vi "test_Bitfile Reload_Simple Scalar to Speciality IO Data type Change.vi"(8 "error in (no error)":errorcluster, 11 "TestCase in":refnum<class "FPGA Addon Bitfile Reload Unit Tests.lvclass">=refnum) -> (0 "error out":errorcluster, 3 "TestCase out":refnum<class "FPGA Addon Bitfile Reload Unit Tests.lvclass">)   [LabVIEW 2026, in "FPGA Addon Bitfile Reload Unit Tests.lvclass"]
uses:
  FPGA Addon Bitfile Reload Unit Tests.lvclass
  APIs/Scripting API/TypeDefs/Output Scalar Data.ctl
  APIs/Scripting API/Scripting API.lvlib
  FPGA Addon Test Class/FPGA Addon Test Class.lvclass
  Addon/Addon System Explorer/FPGA Addon System Explorer.lvlib
  APIs/Scripting API/Public/Bitfile Resources/Import Bitfile Scalars (Instances)/Import Scalars - all.vi
  Addon/Addon Shared/Types/FPGA Addon Data Type.ctl
  Addon/Addon Shared/FPGA Addon Shared.lvlib
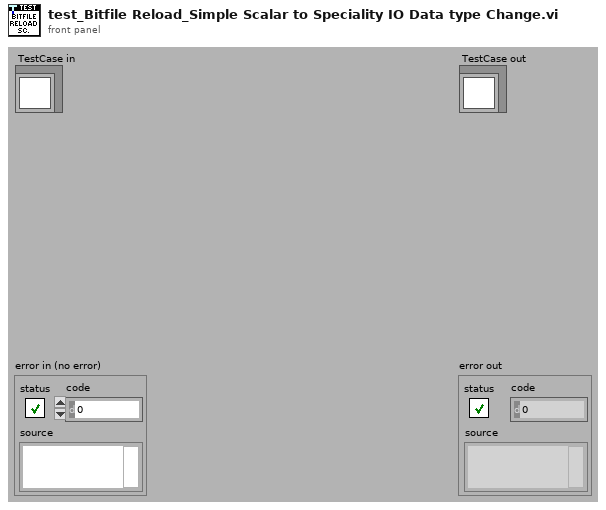
[diagram p1: front panel]
types:
  T1 = typedef "Scripting API.lvlib/Output Scalar Data.ctl" = cluster{"Bitfile Name":string, "SysDef Channel Name":string, "Imported":bool, "Data Type":T2}
  T2 = typedef "FPGA Addon Shared.lvlib/FPGA Addon Data Type.ctl" = enum8{"<Null>", "I8", "I16", "I32", "I64", "U8", "U16", "U32", "U64", "SGL", "Boolean", "Analog PWM In Settings", "Analog PWM In", "Digital PWM In Settings", "Digital PWM In", "Digital PWM Out", "Sine Out", "FXP", "FXP+/-24.5", "FXP+/-16.5", "FXP+/-32.8", "FXP+/-64.32", "FXP+/-16.7", "FXP+/-20.5", "FXP+/-27.5", "FXP+/-32.16", "FXP+16.3", "FXP+18.3", "Digital Static In", "Digital Static Out", "Digital Static In Settings", "Digital WSS Out", "Quad Encoder Settings", "Quad Encoder In", "Group"}
  T3 = typedef "Custom Device API.lvlib/Custom Device Item Ref.ctl" = u64
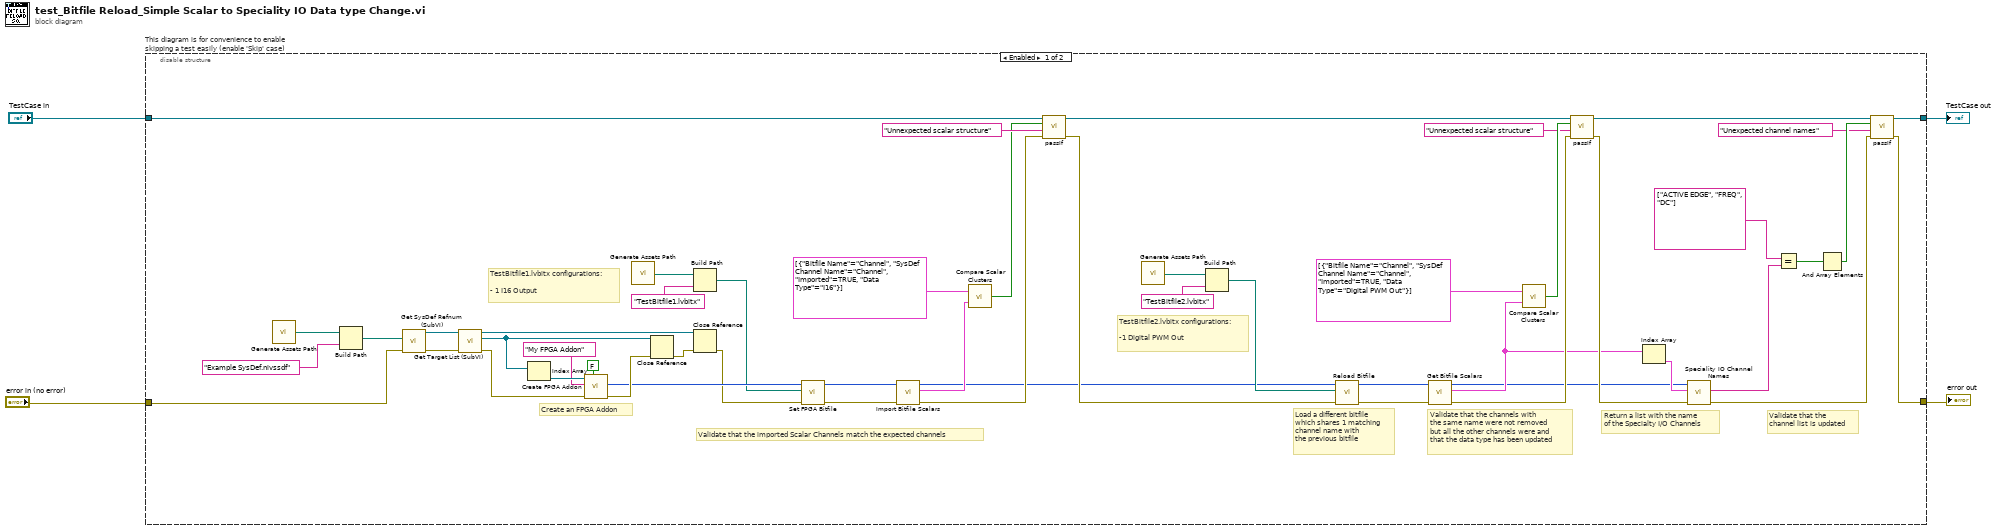
[diagram p0: block diagram]
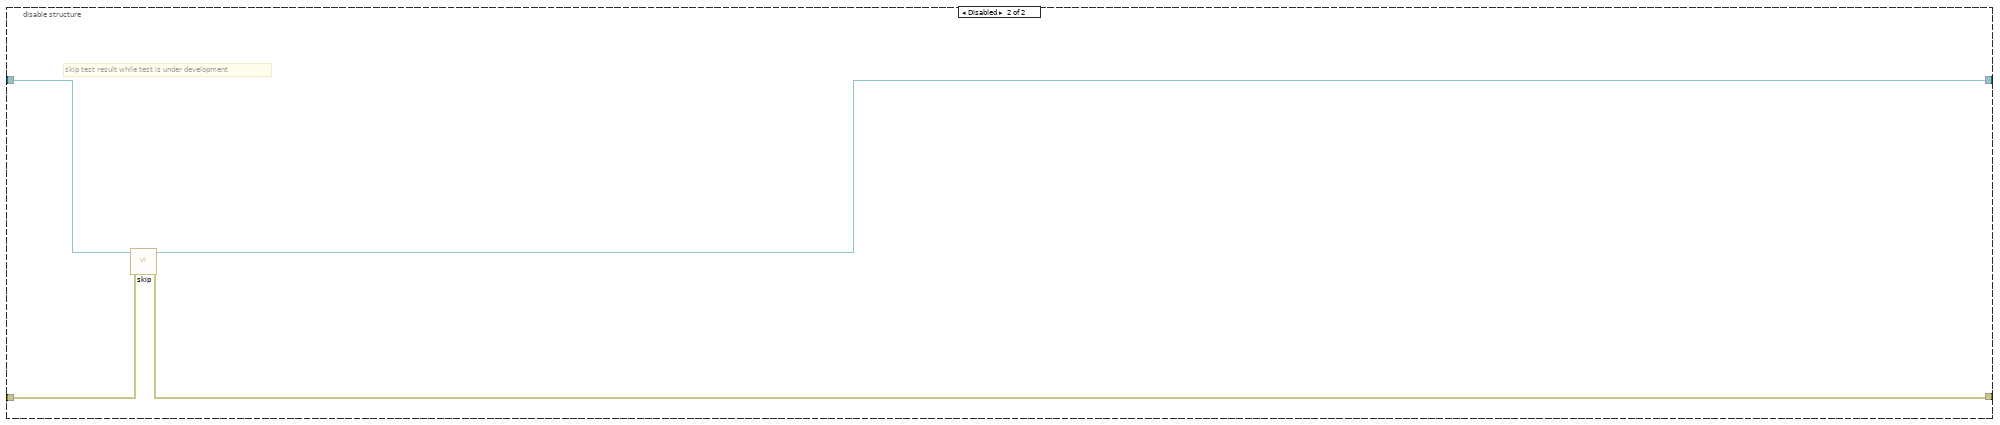
[diagram p2: hidden frame]
diagram:
  n1 = disable-structure "This diagram is for convenience to enable skipping a test easily (enable 'Skip' case)" shown="Enabled" {
    disable-tunnel: "TestCase in" -> [w25 w60]
    disable-tunnel: [w7 w58] -> w1
    disable-tunnel: [w8 w59] -> w3
    disable-tunnel: "error in (no error)" -> [w24 w57]
    frame Enabled {
      # "Validate that the\nchannel list is updated"
      # "Return a list with the name \nof the Specialty I/O Channels"
      # "TestBitfile2.lvbitx configurations:\n\n-1 Digital PWM Out"
      # "TestBitfile1.lvbitx configurations:\n\n- 1 I16 Output"
      # "Validate that the channels with \nthe same name were not removed\nbut all the other channels were and\nthat the data type has been updated"
      # "Load a different bitfile\nwhich shares 1 matching\nchannel name with \nthe previous bitfile"
      # "Validate that the imported Scalar Channels match the expected channels"
      # "Create an FPGA Addon"
      n2 = call "Generate Assets Path.vi"() -> ("Assets path"=w36:path)
      n3 = Build Path(base path=w36, name or relative path="Example SysDef.nivssdf") -> (appended path=w55:path)
      n4 = call "Get SysDef Refnum (SubVI).vi"("error in (no error)"=w24, "System Definition path"=w55) -> ("error out"=w51:errorcluster, "NationalInstruments.VeriStand.SystemDefinitionAPI.SystemDefinition"=w54:refnum<k39>)  [unwired: 8 in]
      n5 = call "Get Target List (SubVI).vi"("error in (no error)"=w51, "NationalInstruments.VeriStand.SystemDefinitionAPI.SystemDefinition"=w54) -> ("error out"=w50:errorcluster, "Target List Refnums"=w49:refnum<k39>[], "NationalInstruments.VeriStand.SystemDefinitionAPI.SystemDefinition"=w48:refnum<k39>)  [unwired: 7 in]
      n6 = Index Array(array=w49) -> (element=w53:refnum<k39>)  [unwired: 1 in]
      n7 = call "Create FPGA Addon.vi"("group scalars"=FALSE, "error in"=w50, "FPGA addon name"="My FPGA Addon", "NationalInstruments.VeriStand.SystemDefinitionAPI.Target"=w53) -> ("error out"=w46:errorcluster, "FPGA addon refnum"=w44:T3)  [unwired: 5 in, 1 out]
      n8 = call "Generate Assets Path.vi"() -> ("Assets path"=w35:path)
      n9 = Close Reference(reference=w49, error in (no error)=w46) -> (error out=w47:errorcluster)
      n10 = Build Path(base path=w35, name or relative path="TestBitfile1.lvbitx") -> (appended path=w41:path)
      n11 = Close Reference(reference=w48, error in (no error)=w47) -> (error out=w43:errorcluster)
      n12 = call "Set FPGA Bitfile.vi"("error in"=w43, "FPGA bitfile path"=w41, "FPGA addon refnum in"=w44) -> ("error out"=w40:errorcluster, "FPGA addon refnum out"=w39:T3)  [unwired: 7 in]
      n13 = call-poly "Import Bitfile Scalars.vi"("error in"=w40, "FPGA addon refnum in"=w39) -> ("error out"=w38:errorcluster, "imported bitfile scalars out"=w21:T1[], "FPGA addon refnum out"=w20:T3)  [unwired: 7 in]
      n14 = call "Compare Scalar Clusters.vi"("Target bitfile scalars in"=w21, "Reference bitfile scalars in"=T1[] [{"Bitfile Name"="Channel", "SysDef Channel Name"="Channel", "Imported"=TRUE, "Data Type"=enum."I16"}] ("imported bitfile scalars out")) -> ("Equal ?"=w34:bool)
      n15 = call-dynamic "passIf.vi"("error in (no error)"=w38, "message (\"\")"="Unnexpected scalar structure" ("message (\"\")"), "pass"=w34, "TestCase in"=w25) -> ("error out"=w22:errorcluster, "TestCase out"=w19:refnum<class "FPGA Addon Bitfile Reload Unit Tests.lvclass">)  [unwired: 6 in]
      n16 = call "Generate Assets Path.vi"() -> ("Assets path"=w32:path)
      n17 = Build Path(base path=w32, name or relative path="TestBitfile2.lvbitx") -> (appended path=w31:path)
      n18 = call "Reload Bitfile.vi"("error in (no error)"=w22, "NewVal"=w31, "Item Ref in"=w20) -> ("error out"=w30:errorcluster, "Section Ref out"=w29:T3)  [unwired: 7 in]
      n19 = call "Get Bitfile Scalars.vi"("error in"=w30, "FPGA addon refnum in"=w29) -> ("error out"=w28:errorcluster, "bitfile scalars out"=w9:T1[], "FPGA addon refnum out"=w6:T3)  [unwired: 7 in]
      n20 = call "Compare Scalar Clusters.vi"("Target bitfile scalars in"=w9, "Reference bitfile scalars in"=T1[] [{"Bitfile Name"="Channel", "SysDef Channel Name"="Channel", "Imported"=TRUE, "Data Type"=enum."Digital PWM Out"}] ("bitfile scalars out")) -> ("Equal ?"=w27:bool)
      n21 = call-dynamic "passIf.vi"("error in (no error)"=w28, "message (\"\")"="Unnexpected scalar structure" ("message (\"\")"), "pass"=w27, "TestCase in"=w19) -> ("error out"=w10:errorcluster, "TestCase out"=w11:refnum<class "FPGA Addon Bitfile Reload Unit Tests.lvclass">)  [unwired: 6 in]
      n22 = Index Array(array=w9) -> (element=w18:T1)  [unwired: 1 in]
      n23 = call "Speciality IO Channel Names.vi"("error in (no error)"=w10, "channel in"=w18, "FPGA Addon ref in"=w6) -> ("error out"=w17:errorcluster, "channel names out"=w16:string[])  [unwired: 6 in, 1 out]
      n24 = Equal?(x=string[] ["ACTIVE EDGE", "FREQ", "DC"], y=w16) -> (x = y?=w14:bool[])
      n25 = And Array Elements(Boolean array=w14) -> (logical AND=w13:bool)
      n26 = call-dynamic "passIf.vi"("error in (no error)"=w17, "message (\"\")"="Unexpected channel names" ("message (\"\")"), "pass"=w13, "TestCase in"=w11) -> ("error out"=w8:errorcluster, "TestCase out"=w7:refnum<class "FPGA Addon Bitfile Reload Unit Tests.lvclass">)  [unwired: 6 in]
    }
    frame Disabled {
      # "skip test result while test is under development"
      n27 = call <vilib>:"skip.vi"("error in (no error)"=w57, "TestCase in"=w60) -> ("error out"=w59:errorcluster, "TestCase out"=w58:refnum<class "FPGA Addon Bitfile Reload Unit Tests.lvclass">)  [unwired: 8 in]
    }
  }
  "error out" <- w3
  "TestCase out" <- w1
